vi "Get AI StringsAndValues.vi"(8 "error in (no error)":errorcluster, 11 "Configuration.DAQ":T1 {"AO terminal config" items=[""=-1, "differential"=10106, "pseudodifferential"=12529]; "AI terminal config" items=[""=-1, "differential"=10106, "pseudodifferential"=12529]; "AI.Coupling" items=[""=0, "AC"=10045, "DC"=10050, "GND"=10066]}) -> (0 "error out":errorcluster, 1 "Values":i32[](array[numeric]), 2 "Strings":string[](array[string]))   [LabVIEW 2019, in "Instrument.Lockin.lvlib" / "Instrument UI.Lockin.lvclass"]
uses:
  Instrument UI.Lockin.lvclass
  Instrument.DAQ/Typedefs/DAQ.Configuration--Cluster--Array.ctl
  Instrument.DAQ/Typedefs/DAQ.Configuration--Cluster.ctl
  Instrument.DAQ/Typedefs/DAQ.Config.AO.Range--enum.ctl
  Instrument.DAQ/Typedefs/DAQ.Config.AI.Range--enum.ctl
  Instrument.DAQ/Typedefs/DAQ.Config.AI.Coupling--enum.ctl
  Instrument.DAQ/Typedefs/DAQ.TerminalConfiguration--ring.ctl
  Instrument.DAQ/Instrument.DAQ.lvclass
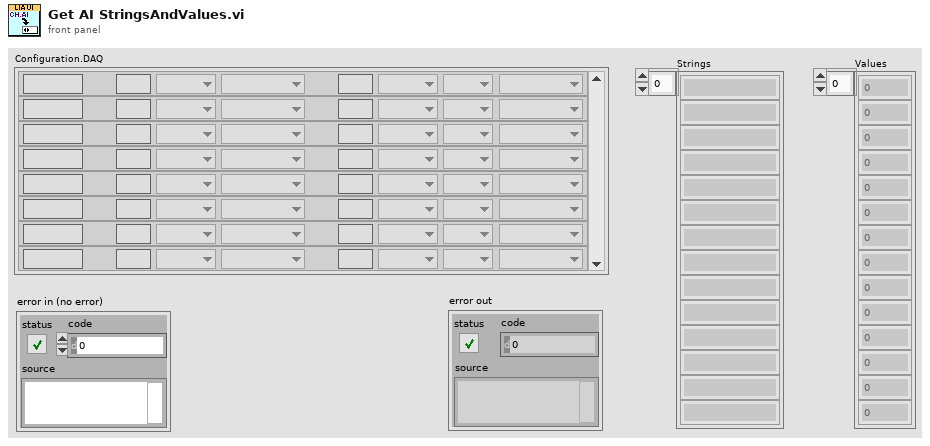
[diagram p1: front panel]
types:
  T1 = typedef "Instrument.Lockin.lvlib/Instrument.DAQ.lvclass/DAQ.Configuration--Cluster--Array.ctl" = T2[]
  T2 = typedef "Instrument.Lockin.lvlib/Instrument.DAQ.lvclass/DAQ.Configuration--Cluster.ctl" = cluster{"Device":string, "AO.Ch":string, "AO.Range":T3, "AI.Ch":string, "AI.Range":T4, "AI.Coupling":T5, "AI terminal config":T6, "AO terminal config":T6}
  T3 = typedef "Instrument.Lockin.lvlib/Instrument.DAQ.lvclass/DAQ.Config.AO.Range--enum.ctl" = enum16{"±0.1", "±1.0", "±10.0", ""}
  T4 = typedef "Instrument.Lockin.lvlib/Instrument.DAQ.lvclass/DAQ.Config.AI.Range--enum.ctl" = enum16{"±0.316", "±1.00", "±3.16", "±10.0", "±31.6", "±42.4", ""}
  T5 = typedef "Instrument.Lockin.lvlib/Instrument.DAQ.lvclass/DAQ.Config.AI.Coupling--enum.ctl" = u16
  T6 = typedef "Instrument.Lockin.lvlib/Instrument.DAQ.lvclass/DAQ.TerminalConfiguration--ring.ctl" = i32
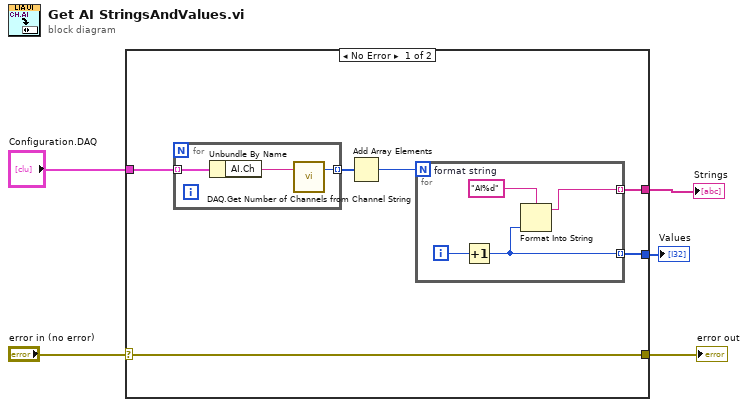
[diagram p0: block diagram]
diagram:
  n1 = case shown="No Error" "error in (no error)" {
    selector: "error in (no error)" -> [w10 w19]
    tunnel: [w10 w19] -> w4
    tunnel: "Configuration.DAQ" -> [w8 _]
    tunnel: [w7 _] -> w2
    tunnel: [w6 _] -> w1
    frame No Error {
      n2 = for {
        tunnel: w8 -> [w14] mode=indexing
        tunnel: [w13] -> w11 mode=indexing
        n3 = Unbundle By Name(w14) -> ("AI.Ch"=w12:string)
        n4 = call "DAQ.Get Number of Channels from Channel String.vi"("Channels String"=w12) -> ("# channels"=w13:i32)  [unwired: 2 in]
      }
      n5 = Add Array Elements(numeric array=w11) -> (sum=w9:i32)
      n6 = for {
        N: w9 -> [_]
        tunnel: [w16] -> w7 mode=indexing
        tunnel: [w15] -> w6 mode=indexing
        i -> [w17]
        w18 = "AI%d"  # format string
        n7 = Increment(x=w17) -> (x+1=w16:i32)
        n8 = Format Into String(format string=w18, w16) -> (resulting string=w15:string)  [unwired: 2 in, 1 out]
      }
    }
    frame Error {
    }
  }
  "error out" <- w4
  "Strings" <- w1
  "Values" <- w2
